vi "Write Color.vi"(8 "error in (no error)":errorcluster, 10 "Color":T1, 11 "ColorSpecification in":refnum<class "ColorSpecification.lvclass">) -> (0 "error out":errorcluster, 3 "ColorSpecification out":refnum<class "ColorSpecification.lvclass">)   [LabVIEW 2018, in "ColorSpecification.lvclass"]
uses:
  ColorSpecification.lvclass
  Product/Color.ctl
  ColorSpecification.lvclass/ColorSpecification.ctl
  Product/Product.lvclass
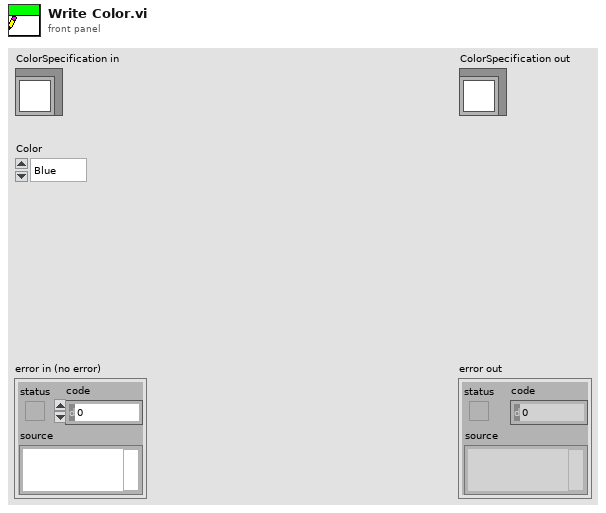
[diagram p1: front panel]
types:
  T1 = typedef "Product.lvclass/Color.ctl" = enum16{"Blue", "Green", "Red"}
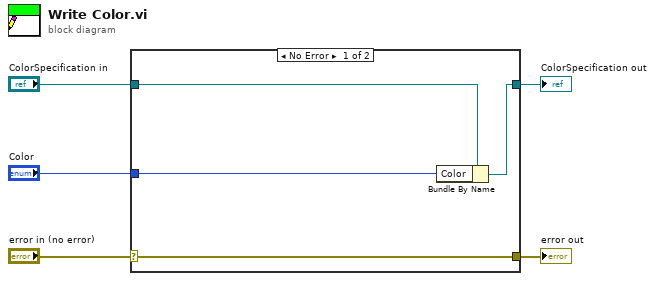
[diagram p0: block diagram]
diagram:
  n1 = case shown="No Error" "error in (no error)" {
    selector: "error in (no error)" -> [w9 w10]
    tunnel: [w9 w10] -> w4
    tunnel: [w7 w11] -> w2
    tunnel: "ColorSpecification in" -> [w8 w11]
    tunnel: "Color" -> [w6 _]
    frame No Error {
      n2 = Bundle By Name(cluster=w8, "Color"=w6) -> (w7:refnum<class "ColorSpecification.lvclass">)
    }
    frame Error {
    }
  }
  "error out" <- w4
  "ColorSpecification out" <- w2
